vi "Make TestCase for Method.vi"(8 "error in (no error)":errorcluster, 10 "Test Method":T1) -> (0 "error out":errorcluster, 3 "LUnit Test Case V2 out":refnum<class "LUnit Test Case V2.lvclass">)   [LabVIEW 2020, in "LUnit Test Case V2 Test Double.lvclass"]
uses:
  LUnit Test Case V2 Test Double.lvclass
  LUnit Test Case/LUnit Test Case V2.lvclass
  Methods.ctl
  LUnit Test Case V2 Test Double.lvclass/LUnit Test Case V2 Test Double.ctl
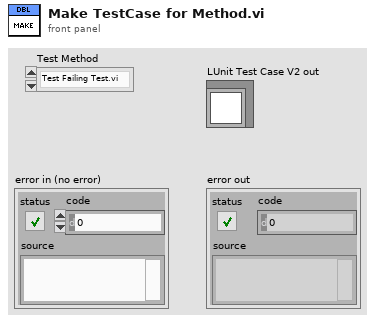
[diagram p1: front panel]
types:
  T1 = typedef "LUnit Test Case V2 Test Double.lvclass/Methods.ctl" = enum16{"Test Failing Test.vi", "Test Passing Test.vi", "Test Error Test.vi", "Test Skip Test.vi", "Test Passing Pass If Test.vi", "Test Failing Pass If Test.vi", "Test Failing Fail If Test.vi", "Test Passing Fail If Test.vi", "Test Passing Pass If Error Test.vi", "Test Failing Pass If Error Test.vi", "Test Passing Fail If Error Test.vi", "Test Failing Fail If Error Test.vi", "Test Passing Pass If Equal Test.vi", "Test Failing Pass If Equal Test.vi", "Test Failing Fail If Equal Test.vi", "Test Passing Fail If Equal Test.vi"}
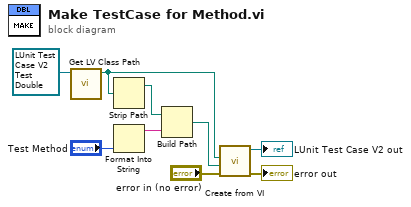
[diagram p0: block diagram]
diagram:
  n1 = call <vilib>:"Get LV Class Path.vi"("object"=refnum<class "LUnit Test Case V2 Test Double.lvclass"> refnum ("LUnit Test Case V2 Test Double.lvclass")) -> ("class path"=w4:path)  [unwired: 9 in, 1 out]
  n2 = Strip Path(path=w4) -> (stripped path=w3:path)  [unwired: 1 out]
  n3 = Format Into String("Test Method") -> (resulting string=w2:string)  [unwired: 3 in, 1 out]
  n4 = Build Path(base path=w3, name or relative path=w2) -> (appended path=w9:path)
  n5 = call "Create from VI.vi"("error in (no error)"="error in (no error)", "Test Method VI Path"=w9, "Test Case LVCLass Path"=w4) -> ("error out"=→"error out":errorcluster, "LUnit Test Case V2 out"=→"LUnit Test Case V2 out":refnum<class "LUnit Test Case V2.lvclass">)  [unwired: 7 in]
